vi "Auto Configure DAQ.vi"(8 "error in (no error)":errorcluster, 11 "DAQmx in":refnum<class "DAQmx.lvclass">) -> (0 "error out":errorcluster, 1 "Configuration.AO":T1 {"output terminal configuration" items=[""=-1, "Differential"=10106, "Pseudodifferential"=12529]}, 2 "Configuration.AI":T5 {"input terminal configuration" items=[""=-1, "Differential"=10106, "Pseudodifferential"=12529]; "Coupling" items=[""=0, "AC"=10045, "DC"=10050, "GND"=10066]}, 3 "DAQmx out":refnum<class "DAQmx.lvclass">, 5 "Devices":T9[](array[typedef]))   [LabVIEW 2019, in "DAQmx.lvclass"]
uses:
  DAQmx.lvclass
  typedefs/DeviceInfo--Cluster.ctl
  typedefs/DAQ.Config.AI--Cluster--Array.ctl
  typedefs/DAQ.Config.AI--Cluster.ctl
  typedefs/DAQ.Config.AI.Coupling--enum.ctl
  typedefs/DAQ.Config.AI.Range--enum.ctl
  typedefs/DAQ.Config.Device Type--enum.ctl
  typedefs/DAQ.Config.AO--Cluster--Array.ctl
  typedefs/DAQ.Config.AO--Cluster.ctl
  typedefs/DAQ.Config.AO.Range--enum.ctl
  DAQmx.lvclass/DAQmx.ctl
  <resource>/objmgr/daqmx.rc
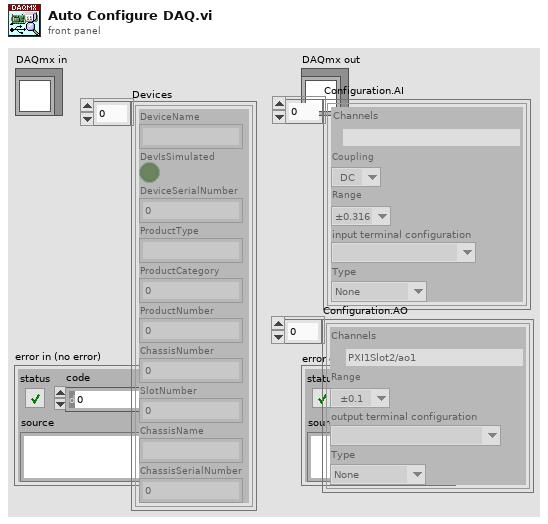
[diagram p1: front panel]
types:
  T1 = typedef "DAQmx.lvclass/DAQ.Config.AO--Cluster--Array.ctl" = T2[]
  T2 = typedef "DAQmx.lvclass/DAQ.Config.AO--Cluster.ctl" = cluster{"Channels":tag, "Range":T3, "output terminal configuration":i32, "Type":T4}
  T3 = typedef "DAQmx.lvclass/DAQ.Config.AO.Range--enum.ctl" = enum16{"±0.1", "±1.0", "±10.0", ""}
  T4 = typedef "DAQmx.lvclass/DAQ.Config.Device Type--enum.ctl" = enum16{"None", "USB-4431", "PXI-446x"}
  T5 = typedef "DAQmx.lvclass/DAQ.Config.AI--Cluster--Array.ctl" = T6[]
  T6 = typedef "DAQmx.lvclass/DAQ.Config.AI--Cluster.ctl" = cluster{"Channels":tag, "Coupling":T7, "Range":T8, "input terminal configuration":i32, "Type":T4}
  T7 = typedef "DAQmx.lvclass/DAQ.Config.AI.Coupling--enum.ctl" = u16
  T8 = typedef "DAQmx.lvclass/DAQ.Config.AI.Range--enum.ctl" = enum16{"±0.316", "±1.00", "±3.16", "±10.0", "±31.6", "±42.4", ""}
  T9 = typedef "DAQmx.lvclass/DeviceInfo--Cluster.ctl" = cluster{"DeviceName":string, "DevIsSimulated":bool, "DeviceSerialNumber":u32, "ProductType":string, "ProductCategory":i32, "ProductNumber":u32, "ChassisNumber":u32, "SlotNumber":u32, "ChassisName":string, "ChassisSerialNumber":u32}
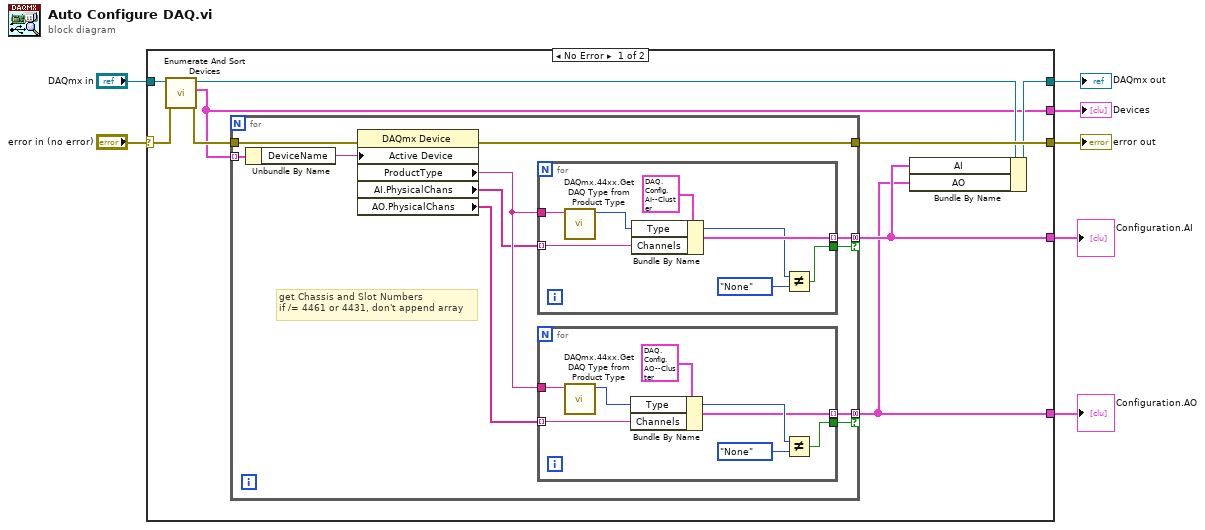
[diagram p0: block diagram]
diagram:
  n1 = case shown="No Error" "error in (no error)" {
    selector: "error in (no error)" -> [w12 w42]
    tunnel: [w16 w42] -> w7
    tunnel: "DAQmx in" -> [w13 w43]
    tunnel: [w15 w43] -> w5
    tunnel: [w10 _] -> w3
    tunnel: [w9 _] -> w2
    tunnel: [w8 _] -> w1
    frame No Error {
      n2 = call "Enumerate And Sort Devices.vi"("error in (no error)"=w12, "DAQmx in"=w13) -> ("error out"=w11:errorcluster, "Devices (sorted)"=w10:T9[], "DAQmx out"=w14:refnum<class "DAQmx.lvclass">)  [unwired: 7 in]
      n3 = for {
        tunnel: [w19] -> w16
        tunnel: [w27] -> w9 mode=concatenating if=w26
        tunnel: w11 -> [w25]
        tunnel: w10 -> [w24] mode=indexing
        tunnel: [w21] -> w8 mode=concatenating if=w20
        # "get Chassis and Slot Numbers\nif /= 4461 or 4431, don't append array"
        n4 = Unbundle By Name(w24) -> ("DeviceName"=w23:string)
        n5 = property class="DAQmx Device"(error in=w25, "Active Device"=w23) -> (error out=w19:errorcluster, "ProductType"=w22:string, "AI.PhysicalChans"=w17:tag[], "AO.PhysicalChans"=w18:tag[])  [unwired: 1 in, 1 out]
        n6 = for {
          tunnel: [w34] -> w27 mode=indexing
          tunnel: w22 -> [w30]
          tunnel: [w29] -> w26
          tunnel: w17 -> [w31] mode=indexing
          n7 = call "DAQmx.44xx.Get DAQ Type from Product Type.vi"("ProductType"=w30) -> ("DAQ Type"=w28:T4)  [unwired: 10 in]
          n8 = Bundle By Name(cluster=T6 {"Channels"="PXI1Slot2/ai0", "Coupling"=10050, "Range"=enum."±0.316", "input terminal configuration"=-1, "Type"=enum."PXI-446x"} ("AI.Config"), "Type"=w28, "Channels"=w31) -> (w34:T6)
          n9 = Not Equal?(x=w28, y=DAQ.Config.Device_Type--enum."None") -> (x != y?=w29:bool)
        }
        n10 = for {
          tunnel: [w36] -> w21 mode=indexing
          tunnel: w22 -> [w41]
          tunnel: [w35] -> w20
          tunnel: w18 -> [w39] mode=indexing
          n11 = call "DAQmx.44xx.Get DAQ Type from Product Type.vi"("ProductType"=w41) -> ("DAQ Type"=w37:T4)  [unwired: 10 in]
          n12 = Bundle By Name(cluster=T2 {"Channels"="PXI1Slot2/ao1", "Range"=enum."±0.1", "output terminal configuration"=-1, "Type"=enum."USB-4431"} ("AO.config"), "Type"=w37, "Channels"=w39) -> (w36:T2)
          n13 = Not Equal?(x=w37, y=DAQ.Config.Device_Type--enum."None") -> (x != y?=w35:bool)
        }
      }
      n14 = Bundle By Name(cluster=w14, "AI"=w9, "AO"=w8) -> (w15:refnum<class "DAQmx.lvclass">)
    }
    frame Error {
    }
  }
  "error out" <- w7
  "DAQmx out" <- w5
  "Devices" <- w3
  "Configuration.AI" <- w2
  "Configuration.AO" <- w1
